vi "section-status-msr.vi"(8 "Boolean":bool, 10 "Enum":enum16{"read", "reset", "add"}(ring)) -> (2 "section.status":bool)   [LabVIEW 2015]
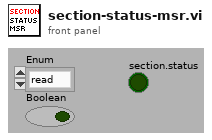
[diagram p1: front panel]
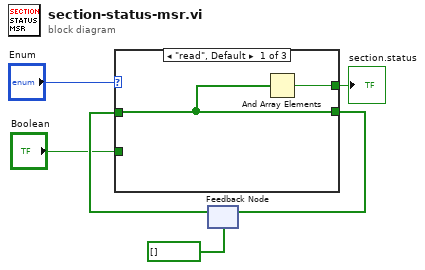
[diagram p0: block diagram]
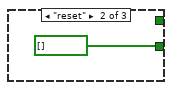
[diagram p2: hidden frame]
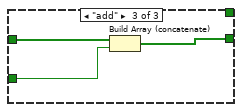
[diagram p3: hidden frame]
diagram:
  n1 = feedback #1(bool[] []) -> (w4:bool[])
  n2 = case shown="\"read\", Default" "Enum" {
    tunnel: w4 -> [w8 _ w12]
    tunnel: [w8 bool[] [] w11] -> w3
    tunnel: "Boolean" -> [_ _ w10]
    tunnel: [w7 _ _] -> w1
    frame "read", Default {
      n3 = And Array Elements(Boolean array=w8) -> (logical AND=w7:bool)
    }
    frame "reset" {
    }
    frame "add" {
      n4 = Build Array (concatenate)(w12, w10) -> (w11:bool[])
    }
  }
  "section.status" <- w1
  n5 = feedback-in #1(w3) -> ()
